vi "Pre-Build VI - Run Unit Tests.vi"(8 "error in (no error)":errorcluster) -> (0 "error out":errorcluster, 1 "VIs without test coverage":string[](array[string]), 2 "error type":enum16{"fatal", "non-fatal", "warning"}(ring))   [LabVIEW 2009]
uses:
  <userlib>/_OpenG.lib/file/file.llb/Build Path - File Names Array__ogtk.vi
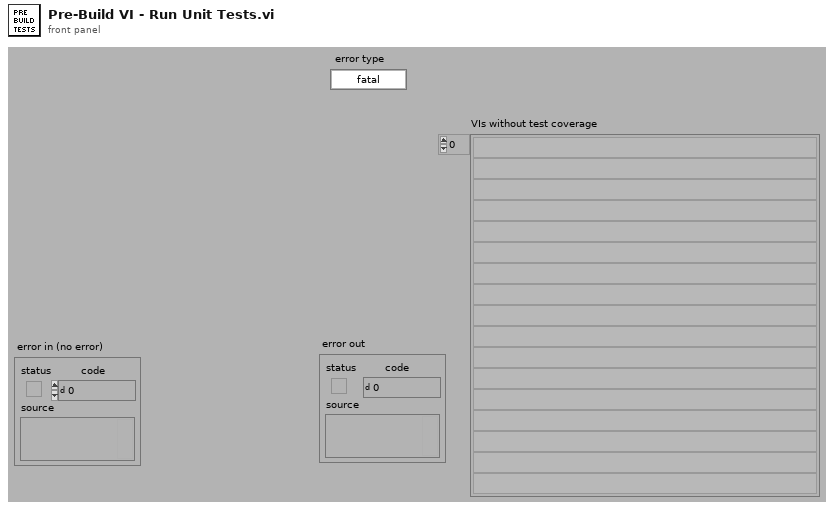
[diagram p1: front panel]
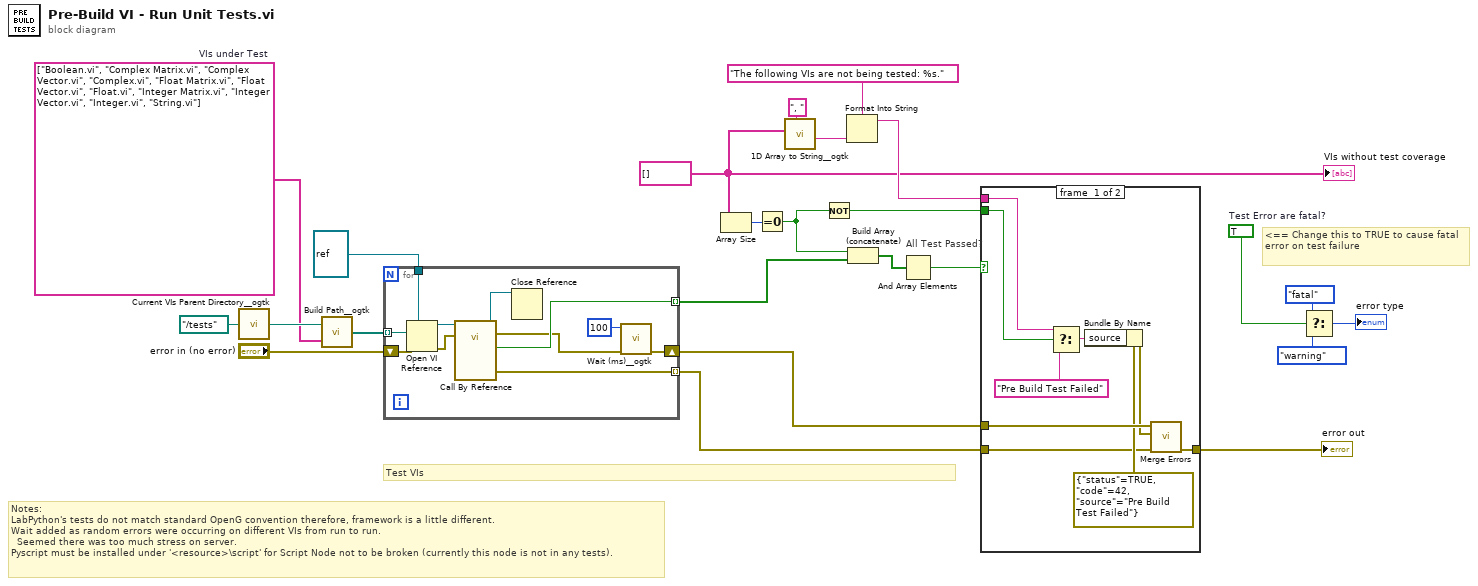
[diagram p0: block diagram]
diagram:
  w1 = string[] [] ("filtered array")
  w4 = string[] ["Boolean.vi", "Complex Matrix.vi", "Complex Vector.vi", "Complex.vi", "Float Matrix.vi", "Float Vector.vi", "Float.vi", "Integer Matrix.vi", "Integer Vector.vi", "Integer.vi", "String.vi"]  # VIs under Test
  w16 = TRUE  # Test Error are fatal?
  # "Notes: \nLabPython's tests do not match standard OpenG convention therefore, framework is a little different.\nWait added as random errors were occurring on different VIs from run to run. \n  Seemed there was too much stress on server.\nPyscript must be installed under '<resource>\\script' for Script Node not to be broken (currently this node is not in any tests)."
  # "<== Change this to TRUE to cause fatal error on test failure"
  # "All Test Passed?"
  # "Test VIs"
  n1 = call <userlib>:"Current VIs Parent Directory__ogtk.vi"("Relative path (.)"=path "../tests") -> ("Parent Directory (+ Relative)"=w5:path)  [unwired: 4 in]
  n2 = call-poly <userlib>:"Build Path__ogtk.vi"("name or relative path"=w4, "base path"=w5) -> ("appended path"=w3:path[])
  n3 = for {
    tunnel: w3 -> [w35] mode=indexing
    tunnel: refnum<vi> refnum ("type specifier VI Refnum (for type only)") -> [w34]
    shift-right: [w26] -> w10
    shift-left: "error in (no error)" -> [w31]
    tunnel: [w30] -> w9 mode=indexing
    tunnel: [w28] -> w8 mode=indexing
    n4 = Open VI Reference(type specifier VI Refnum (for type only)=w34, vi path=w35, error in (no error)=w31) -> (vi reference=w33:refnum<vi>, error out=w32:errorcluster)  [unwired: 3 in]
    n5 = call-by-ref "?"(reference=w33, error in=w32) -> (reference out=w29:refnum<vi>, error out=w27:errorcluster, 0:"error out"=w28:errorcluster, "Passed?"=w30:bool)  [unwired: 10 in]
    n6 = Close Reference(reference=w29) -> ()  [unwired: 1 in, 1 out]
    n7 = call <userlib>:"Wait (ms)__ogtk.vi"("error in (no error)"=w27, "milliseconds to wait"=u32 100) -> ("error out"=w26:errorcluster)  [unwired: 8 in, 1 out]
  }
  n8 = Array Size(array=w1) -> (size(s)=w7:i32)
  n9 = Equal To 0?(x=w7) -> (x = 0?=w6:bool)
  n10 = call <userlib>:"1D Array to String__ogtk.vi"("delimiter (Tab)"=", ", "Array of Strings"=w1) -> ("delimited string"=w21:string)  [unwired: 9 in]
  n11 = Not(x=w6) -> (.not. x?=w18:bool)
  n12 = Format Into String(format string="The following VIs are not being tested: %s.", w21) -> (resulting string=w19:string)  [unwired: 2 in, 1 out]
  n13 = Build Array (concatenate)(w6, w9) -> (w24:bool[])
  n14 = And Array Elements(Boolean array=w24) -> (logical AND=w23:bool)
  n15 = case shown="False" w23 {
    tunnel: w10 -> [w44 w45]
    tunnel: [w43 w45] -> w17
    tunnel: w18 -> [w42 _]
    tunnel: w19 -> [w41 _]
    tunnel: w8 -> [w36 _]
    frame #0 {
      n16 = Select(t=w41, s=w42, f="Pre Build Test Failed" ("source")) -> (s? t:f=w39:string)
      n17 = Bundle By Name(cluster=errorcluster {"status"=TRUE, "code"=42, "source"="Pre Build Test Failed"} ("error out"), "source"=w39) -> (w38:errorcluster)
      n18 = call <vilib>:"Merge Errors.vi"("error array in"=w36, "error in 2 (no error)"=w38, "error in 1 (no error)"=w44) -> ("error out"=w43:errorcluster)  [unwired: 4 in]
    }
    frame #1 {
    }
  }
  "error out" <- w17
  n19 = Select(t=enum16{"fatal", "non-fatal", "warning"}."fatal" ("error type"), s=w16, f=enum16{"fatal", "non-fatal", "warning"}."warning" ("error type")) -> (s? t:f=→"error type":enum16{"fatal", "non-fatal", "warning"})
  "VIs without test coverage" <- w1
